vi "XY Graph Replace N Plots Helper Function.vi"(8 "error in (no error)":errorcluster, 9 "Replaced Plots Indices (last plots)":i32[](array[numeric]), 10 "Array of Plots":cluster{"X Array":dbl[], "Y Array":dbl[]}[](array[cluster]), 11 "Current Plots":cluster{"X Array":dbl[], "Y Array":dbl[]}[](array[cluster])) -> (0 "error out":errorcluster, 1 "Replaced Plots Indices":i32[](array[numeric]), 3 "New Plots":cluster{"X Array":dbl[], "Y Array":dbl[]}[](array[cluster]))   [LabVIEW 2021, in "XY Graph Add-Ons.lvlib"]
uses:
  XY Graph Add-Ons.lvlib
  <userlib>/_Hooovahh/Array VIMs/Controls/Enum - Order Ascending Descending.ctl
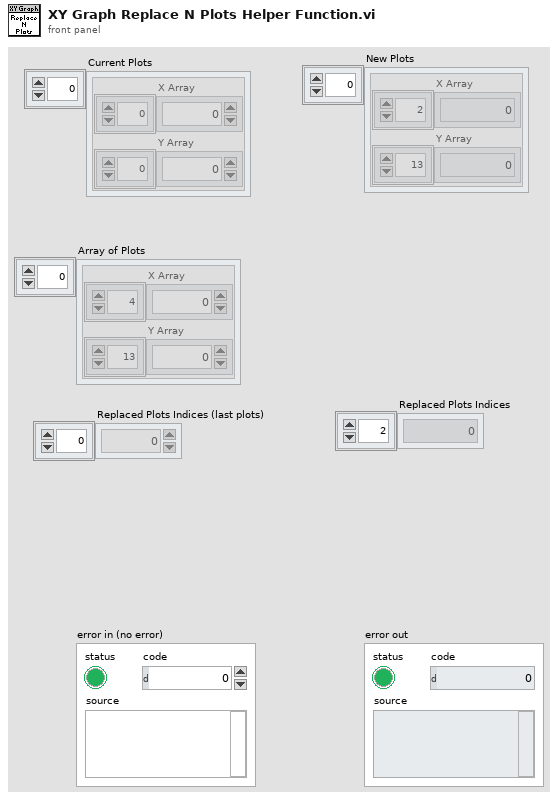
[diagram p1: front panel]
types:
  T1 = typedef "Enum - Order Ascending Descending.ctl" = enum16{"Ascending", "Descending"}
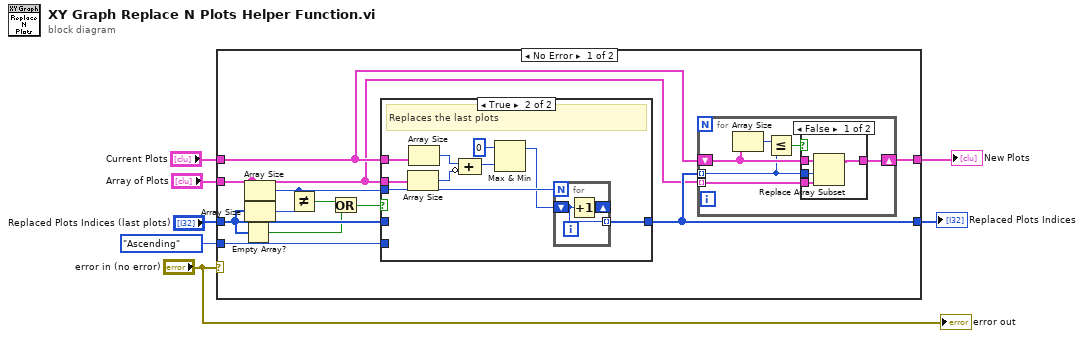
[diagram p0: block diagram]
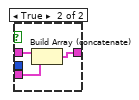
[diagram p2: hidden frame]
diagram:
  n1 = case shown="No Error" "error in (no error)" {
    tunnel: "Replaced Plots Indices (last plots)" -> [w16 _]
    tunnel: "Array of Plots" -> [w8 _]
    tunnel: Enum_-_Order_Ascending_Descending."Ascending" ("Order (Ascending)") -> [w18 _]
    tunnel: "Current Plots" -> [w9 w44]
    tunnel: [w11 w44] -> w3
    tunnel: [w10 _] -> w2
    frame No Error {
      n2 = Empty Array?(array=w16) -> (empty?=w14:bool)
      n3 = Array Size(array=w8) -> (size(s)=w12:i32)
      n4 = Array Size(array=w16) -> (size(s)=w17:i32)
      n5 = Not Equal?(x=w12, y=w17) -> (x != y?=w15:bool)
      n6 = Or(x=w15, y=w14) -> (x .or. y?=w13:bool)
      n7 = case shown="True" w13 {
        tunnel: w8 -> [_ w38]
        tunnel: w18 -> [_ _]
        tunnel: w9 -> [_ w39]
        tunnel: w16 -> [w32 _]
        tunnel: [w32 w33] -> w10
        tunnel: w12 -> [_ w37]
        frame False {
          # "plots are assumed sorted"
        }
        frame True {
          # "Replaces the last plots"
          n8 = Array Size(array=w38) -> (size(s)=w40:i32)
          n9 = Array Size(array=w39) -> (size(s)=w41:i32)
          n10 = Compound Arithmetic op=ADD(w41, invert w40) -> (w35:i32)
          n11 = Max & Min(x=0, y=w35) -> (max(x,y)=w36:i32)  [unwired: 1 out]
          n12 = for {
            N: w37 -> [_]
            shift-right: [w43] -> _
            shift-left: w36 -> [w42]
            tunnel: [w42] -> w33 mode=indexing
            n13 = Increment(x=w42) -> (x+1=w43:i32)
          }
        }
      }
      n14 = for {
        shift-right: [w24] -> w11
        shift-left: w9 -> [w21]
        tunnel: w10 -> [w20] mode=indexing
        tunnel: w8 -> [w23] mode=indexing
        n15 = Array Size(array=w21) -> (size(s)=w22:i32)
        n16 = Less Or Equal?(x=w22, y=w20) -> (x <= y?=w19:bool)
        n17 = case shown="False" w19 {
          tunnel: [w28 w30] -> w24
          tunnel: w23 -> [w27 w29]
          tunnel: w21 -> [w26 w31]
          tunnel: w20 -> [w25 _]
          frame False {
            n18 = Replace Array Subset(array=w26, new element=w27, index=w25) -> (w28:cluster{"X Array":dbl[], "Y Array":dbl[]}[])
          }
          frame True {
            n19 = Build Array (concatenate)(w31, w29) -> (w30:cluster{"X Array":dbl[], "Y Array":dbl[]}[])
          }
        }
      }
    }
    frame Error {
    }
  }
  "New Plots" <- w3
  "Replaced Plots Indices" <- w2
  "error out" <- "error in (no error)"
